vi "SPI Commands Microphone ADC.vi"(7 "Chip Select":u8, 9 "Data to Device":u64=2147483648 format="%b", 10 "SPI PHY Settings":T1={"Divide Value"=10, "Transfer Length (bits)"=16, "CS Asserted Polarity"=FALSE, "Clock Polarity (CPOL)"=FALSE, "Clock Phase (CPHA)"=FALSE, "Lengthen MISO Setup"=FALSE, "Direction Change Bit"=0, "MOSI Starts as Output"=FALSE, "Tristatable MOSI"=FALSE} {"Direction Change Bit" max=64 step=1; "Transfer Length (bits)" min=1 max=64 step=1}, 11 "SPI API References":T2) -> (2 "Data from Device":u64)   [LabVIEW 2014]
uses:
  <vilib>/SPI API/SPIAPI/Controls/Internal Data (SPI API).ctl
  <userlib>/_NI SPI IP/FPGA/Controllers/Public/Transfer Settings.ctl
  <vilib>/Platform/TimedLoop/XDataNode/timing_clust.ctl
  <vilib>/Platform/TimedLoop/XDataNode/nitl_modes.ctl
  <vilib>/Platform/TimedLoop/XDataNode/wakeup.ctl
  <vilib>/rvi/Emulation/niFpgaGetClockAttributes.vi
  <vilib>/rvi/Emulation/niFpgaSctlEmulationGetInTimedLoop.vi
  <vilib>/rvi/Emulation/niFpgaEmulationReportErrorSimple.vi
  <vilib>/rvi/Emulation/niFpgaCriticalErrorInLSC.vi
  <vilib>/Platform/TimedLoop/XDataNode/XDataNode.xnode
  <vilib>/Platform/TimedLoop/XDataNode/XDNodeRunTimeDep.lvlib
  <userlib>/_NI SPI IP/FPGA/Controllers/NI SPI IP FPGA.lvlib
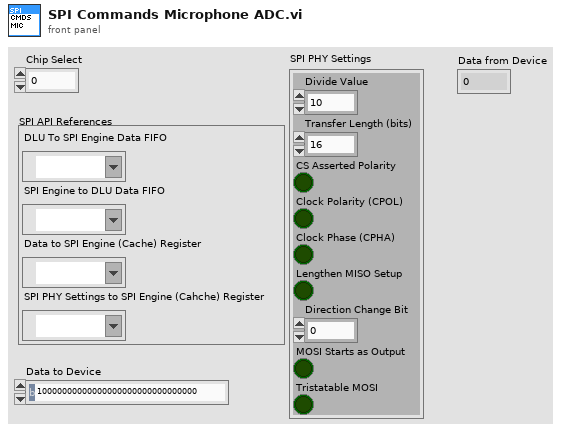
[diagram p1: front panel]
types:
  T1 = typedef "NI SPI IP FPGA.lvlib/Transfer Settings.ctl" = cluster{"Divide Value":u8, "Transfer Length (bits)":u8, "CS Asserted Polarity":bool, "Clock Polarity (CPOL)":bool, "Clock Phase (CPHA)":bool, "Lengthen MISO Setup":bool, "Direction Change Bit":u8, "MOSI Starts as Output":bool, "Tristatable MOSI":bool}
  T2 = typedef "Internal Data (SPI API).ctl" = cluster{"DLU To SPI Engine Data FIFO":refnum<k21>, "SPI Engine to DLU Data FIFO":refnum<k21>, "Data to SPI Engine (Cache) Register":refnum<k21>, "SPI PHY Settings to SPI Engine (Cahche) Register":refnum<k21>}
  T3 = typedef "XDNodeRunTimeDep.lvlib/timing_clust.ctl" = cluster{"Expected End [f-1]":u64, "Actual End [f-1]":u64, "Finished Late? [f-1]":bool, "Expected End [i-1]":u64, "Actual End [i-1]":u64, "Finished Late? [i-1]":bool, "Expected Start [i]":u64, "Actual Start [i]":u64, "Expected Start [f]":u64, "Actual Start [f]":u64, "Source Name":string, "Structure Name":string, "Period":i64, "Deadline":i64, "Offset":i64, "Start":i64, "Priority":i32, "Timeout":i32, "Mode":T4, "Wakeup Reason":T5, "Error":errorcluster, "Source Type":string, "Secondary Source Type":string, "Global End Time":u64, "Global Start Time":u64, "Frame Duration":u64, "Iteration Duration":u64, "Assigned CPU":i32, "I/O Scan Engine Mode":u32}
  T4 = typedef "XDNodeRunTimeDep.lvlib/nitl_modes.ctl" = enum32{"No Change", "Process missed periods, maintain original phase", "Discard missed periods, maintain original phase", "Process missed periods, ignore original phase", "Discard missed periods, ignore original phase"}
  T5 = typedef "XDNodeRunTimeDep.lvlib/wakeup.ctl" = enum32{"Normal", "Aborted", "Asynchronous wakeup", "Timing source error", "Timed loop error", "Timeout"}
  T6 = typedef "SPI Response Information.ctl" = cluster{"Data to Node":u64, "Node Id":u16}
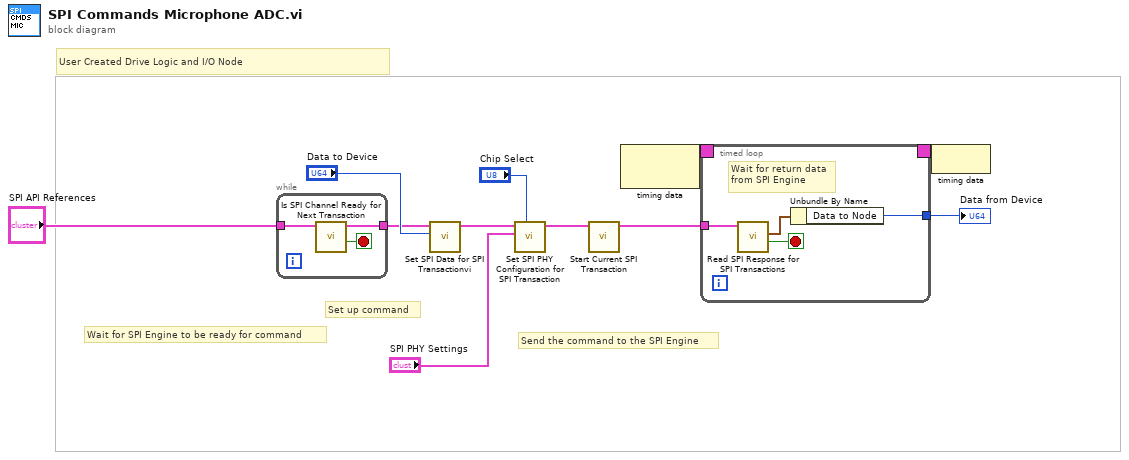
[diagram p0: block diagram]
diagram:
  # "Send the command to the SPI Engine"
  # "Set up command"
  # "Wait for SPI Engine to be ready for command"
  # "User Created Drive Logic and I/O Node"
  n1 = while {
    tunnel: "SPI API References" -> [w13]
    tunnel: [w12] -> w3
    stop <- w14 stop-if-true
    n2 = call <vilib>:"Is SPI Channel Ready for Next Transaction.vi"("Private Data In"=w13) -> ("SPI Channel Ready"=w14:bool, "Private Data Out"=w12:T2)  [unwired: 7 in, 2 out]
  }
  n3 = call <vilib>:"Set SPI Data for SPI Transactionvi.vi"("Data In"="Data to Device", "Private Data In"=w3) -> ("Private Data Out"=w5:T2)  [unwired: 8 in, 1 out]
  n4 = call <vilib>:"Set SPI PHY Configuration for SPI Transaction.vi"("Chip Select"="Chip Select", "SPI PHY Settings"="SPI PHY Settings", "Private Data In"=w5) -> ("Private Data Out"=w7:T2)  [unwired: 7 in, 1 out]
  n5 = call <vilib>:"Start Current SPI Transaction.vi"("Private Data In"=w7) -> ("Private Data Out"=w8:T2)  [unwired: 8 in, 2 out]
  n6 = node-c288() -> (w11:T3)  [unwired: 1 in]
  n7 = timed-loop {
    timing: w11 -> [_]
    timing-out: [_] -> w10
    tunnel: w8 -> [w18]
    tunnel: [w15] -> w1
    stop <- w17 stop-if-true
    # "Wait for return data\nfrom SPI Engine"
    n8 = call <vilib>:"Read SPI Response for SPI Transactions.vi"("Private Data In"=w18) -> ("Read Data Valid?"=w17:bool, "Read Data"=w16:T6)  [unwired: 7 in, 2 out]
    n9 = Unbundle By Name(w16) -> ("Data to Node"=w15:u64)
  }
  "Data from Device" <- w1
  n10 = node-c288(w10) -> ()
